vi "Resize.vi"(4 "Send events? [T]":bool=TRUE, 6 "Defer Panel Updates? [F]":bool, 7 "VI Refnum":refnum<vi>, 8 "error in (no error)":errorcluster, 10 "Bounds":T1, 11 "MMI Scaling in":refnum<class "Object.lvclass">) -> (0 "error out":errorcluster, 2 "Resized":string[](array[string]), 3 "MMI Scaling out":refnum<class "Object.lvclass">)   [LabVIEW 2013, in "Object.lvclass"]
uses:
  Object.lvclass
  <vilib>/Utility/miscctls.llb/LVRectTypeDef.ctl
  Object.lvclass/Object.ctl
  IObject.lvclass
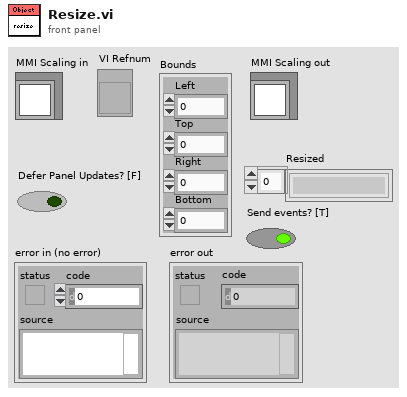
[diagram p1: front panel]
types:
  T1 = typedef "LVRectTypeDef.ctl" = cluster{"Left":i16, "Top":i16, "Right":i16, "Bottom":i16}
  T2 = cluster{"Left":dbl, "Top":dbl, "Right":dbl, "Bottom":dbl}
  T3 = cluster{"Left":i16, "Top":i16, "Left":i16, "Top":i16}
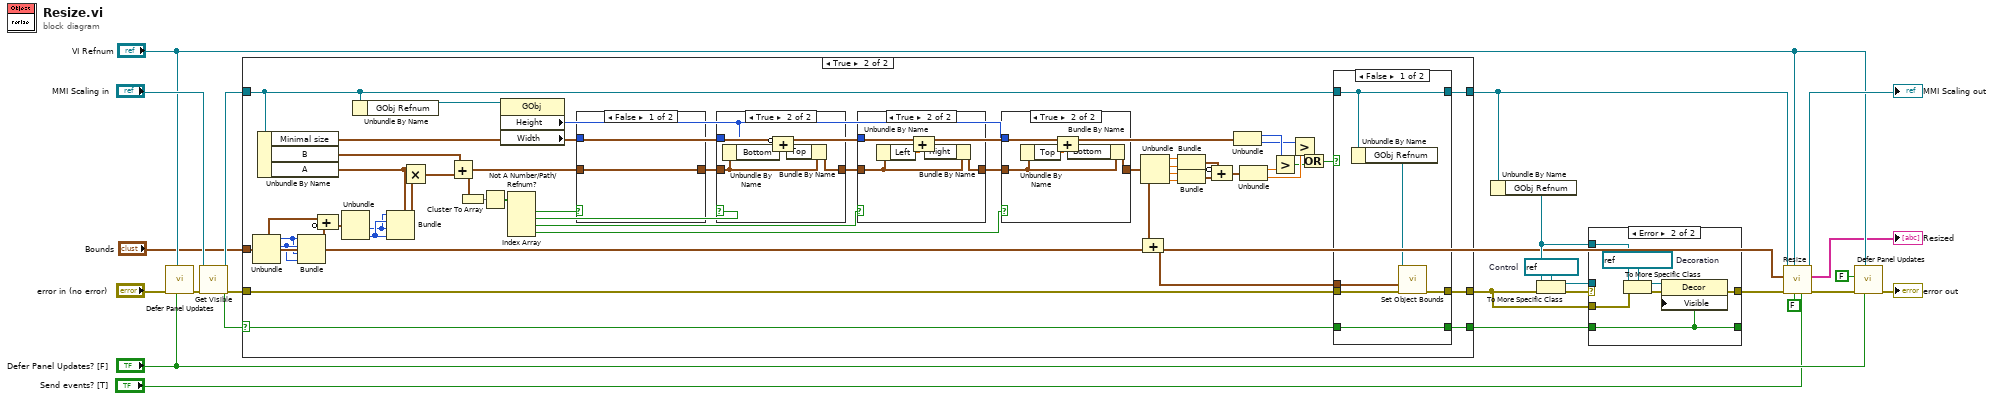
[diagram p0: block diagram]
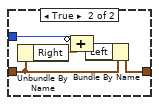
[diagram p6: hidden frame]
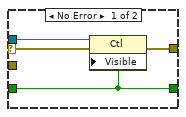
[diagram p8: hidden frame]
diagram:
  w19 = refnum<vi> refnum  # Control
  n1 = call "Defer Panel Updates.vi"("Set Defer Panel Updates? [T]"="Defer Panel Updates? [F]", "VI Refnum"="VI Refnum", "error in (no error)"="error in (no error)") -> ("error out"=w16:errorcluster)  [unwired: 8 in]
  n2 = call-dynamic "Get Visible.vi"("error in (no error)"=w16, "IObject in"="MMI Scaling in") -> ("error out"=w7:errorcluster, "Visible?"=w4:bool, "IObject out"=w14:refnum<class "Object.lvclass">)  [unwired: 6 in, 1 out]
  n3 = case shown="True" w4 {
    selector: w4 -> [w25 w50]
    tunnel: [w26 w74] -> w6
    tunnel: w7 -> [w26 w73]
    tunnel: w14 -> [w27 w43]
    tunnel: [w27 w51] -> w8
    tunnel: "Bounds" -> [_ w62]
    tunnel: [w25 w49] -> w3
    frame False {
    }
    frame True {
      n4 = Unbundle(w62) -> ("Left"=w69:i16, "Top"=w70:i16)  [unwired: 2 out]
      n5 = Unbundle By Name(w43) -> ("Minimal size"=w60:cluster{"Horizontal":i16, "Vertical":i16}, "B"=w61:T2, "A"=w28:T2)
      n6 = Bundle("Left"=w69, "Top"=w70, "Left"=w69, "Top"=w70) -> (w71:T3)  [unwired: 1 in]
      n7 = Compound Arithmetic op=ADD(w62, invert w71) -> (w32:T1)
      n8 = Unbundle(w32) -> ("Right"=w30:i16, "Bottom"=w31:i16)  [unwired: 2 out]
      n9 = Unbundle By Name(w43) -> ("GObj Refnum"=w42:refnum<vi>)
      n10 = Bundle(cluster=w28, "Left"=w30, "Top"=w31, "Right"=w30, "Bottom"=w31) -> (w29:T2)
      n11 = Multiply(x=w28, y=w29) -> (x*y=w72:T2)
      n12 = Add(x=w61, y=w72) -> (x+y=w44:T2)
      n13 = Cluster To Array(cluster=w44) -> (array=w47:dbl[])
      n14 = Not A Number/Path/Refnum?(number/path/refnum=w47) -> (NaN/Path/Refnum?=w46:bool[])
      n15 = property class="GObj"(reference=w42) -> ("Height"=w33:u32, "Width"=w37:u32)  [unwired: 1 in, 2 out]
      n16 = Index Array(array=w46) -> (element #1=w45:bool, element #2=w41:bool, element #3=w39:bool, element #4=w34:bool)  [unwired: 4 in]
      n17 = case shown="False" w45 {
        tunnel: w44 -> [w93 w98]
        tunnel: w37 -> [_ w94]
        tunnel: [w93 w97] -> w38
        frame False {
        }
        frame True {
          n18 = Unbundle By Name(w98) -> ("Right"=w96:dbl)
          n19 = Compound Arithmetic op=ADD(invert w94, w96) -> (w95:dbl)
          n20 = Bundle By Name(cluster=w98, "Left"=w95) -> (w97:T2)
        }
      }
      n21 = case shown="True" w41 {
        tunnel: w38 -> [w87 w92]
        tunnel: [w87 w91] -> w40
        tunnel: w33 -> [_ w88]
        frame False {
        }
        frame True {
          n22 = Unbundle By Name(w92) -> ("Bottom"=w90:dbl)
          n23 = Compound Arithmetic op=ADD(invert w88, w90) -> (w89:dbl)
          n24 = Bundle By Name(cluster=w92, "Top"=w89) -> (w91:T2)
        }
      }
      n25 = case shown="True" w39 {
        tunnel: w40 -> [w81 w86]
        tunnel: [w81 w85] -> w35
        tunnel: w37 -> [_ w83]
        frame False {
        }
        frame True {
          n26 = Unbundle By Name(w86) -> ("Left"=w84:dbl)
          n27 = Compound Arithmetic op=ADD(w83, w84) -> (w82:dbl)
          n28 = Bundle By Name(cluster=w86, "Right"=w82) -> (w85:T2)
        }
      }
      n29 = case shown="True" w34 {
        tunnel: w35 -> [w75 w80]
        tunnel: [w75 w79] -> w36
        tunnel: w33 -> [_ w77]
        frame False {
        }
        frame True {
          n30 = Unbundle By Name(w80) -> ("Top"=w78:dbl)
          n31 = Compound Arithmetic op=ADD(w77, w78) -> (w76:dbl)
          n32 = Bundle By Name(cluster=w80, "Bottom"=w76) -> (w79:T2)
        }
      }
      n33 = Unbundle(w36) -> ("Left"=w63:dbl, "Top"=w64:dbl, "Right"=w65:dbl, "Bottom"=w66:dbl)
      n34 = Compound Arithmetic op=ADD(w36, w71) -> (w48:cluster{"Left":dbl, "Top":dbl, dbl, dbl})
      n35 = Bundle("Left"=w63, "Top"=w64) -> (w67:cluster{"Left":dbl, "Top":dbl})  [unwired: 1 in]
      n36 = Bundle("Right"=w65, "Bottom"=w66) -> (w68:cluster{"Right":dbl, "Bottom":dbl})  [unwired: 1 in]
      n37 = Compound Arithmetic op=ADD(invert w67, w68) -> (w59:cluster{dbl, dbl})
      n38 = Unbundle(w60) -> ("Horizontal"=w57:i16, "Vertical"=w56:i16)
      n39 = Unbundle(w59) -> (w58:dbl, w55:dbl)
      n40 = Greater?(x=w57, y=w58) -> (0:w53:bool)
      n41 = Greater?(x=w56, y=w55) -> (0:w54:bool)
      n42 = Or(x=w54, y=w53) -> (x .or. y?=w52:bool)
      n43 = case shown="False" w52 {
        tunnel: [w104 w105] -> w74
        tunnel: w73 -> [w102 w105]
        tunnel: w43 -> [w100 w106]
        tunnel: w48 -> [w101 _]
        tunnel: [w100 w106] -> w51
        tunnel: w50 -> [w99 _]
        tunnel: [w99 _] -> w49
        frame False {
          n44 = Unbundle By Name(w100) -> ("GObj Refnum"=w103:refnum<vi>)
          n45 = call "Set Object Bounds.vi"("error in (no error)"=w102, "rect"=w101, "GObject"=w103) -> ("error out"=w104:errorcluster)  [unwired: 7 in, 1 out]
        }
        frame True {
        }
      }
    }
  }
  n46 = Unbundle By Name(w8) -> ("GObj Refnum"=w17:refnum<vi>)
  n47 = To More Specific Class(target class=w19, reference=w17, error in=w6) -> (specific class reference=w20:refnum<vi>, error out=w18:errorcluster)
  n48 = case shown="Error" w18 {
    selector: w18 -> [w108 _]
    tunnel: [w110 w117] -> w5
    tunnel: w20 -> [w109 _]
    tunnel: w6 -> [_ w115]
    tunnel: w17 -> [_ w112]
    tunnel: w3 -> [w107 w111]
    tunnel: [w107 w111] -> _
    frame No Error {
      n49 = property class="Ctl"(reference=w109, error in=w108, "Visible"=w107) -> (error out=w110:errorcluster)  [unwired: 1 out]
    }
    frame Error {
      w116 = refnum<vi> refnum  # Decoration
      n50 = To More Specific Class(target class=w116, reference=w112, error in=w115) -> (specific class reference=w113:refnum<vi>, error out=w114:errorcluster)
      n51 = property class="Decor"(reference=w113, error in=w114, "Visible"=w111) -> (error out=w117:errorcluster)  [unwired: 1 out]
    }
  }
  n52 = call-parent "Resize.vi"("Send events? [T]"="Send events? [T]", "Defer Panel Updates? [T]"=FALSE, "VI Refnum"="VI Refnum", "error in (no error)"=w5, "Bounds"="Bounds", "MMI Scaling in"=w8) -> ("error out"=w13:errorcluster, "Resized"=→"Resized":string[], "MMI Scaling out"=→"MMI Scaling out":refnum<class "Object.lvclass">)  [unwired: 3 in]
  n53 = call "Defer Panel Updates.vi"("Set Defer Panel Updates? [T]"="Defer Panel Updates? [F]", "VI Refnum"="VI Refnum", "error in (no error)"=w13, "Defer Panel Updates? [T]"=FALSE) -> ("error out"=→"error out":errorcluster)  [unwired: 7 in]
